vi "Save Bar Sample test results to Disk.vi"(0 "Test Settings":T4={"Current Level"=0.0, "Compliance Level"=0.0, "Soak Time"=0.0, "NPLC Voltmeter"=1.0, "Count Voltmeter"=1, "NPLC Ammeter"=1.0, "Count Ammeter"=1, "Sample Resistivity"=enum."Low", "Sample Thickness"=0.0, "Magnetic Flux"=0.0, "Units"=enum."T", "Sample Dimensions x"=0.0, "Sample Dimensions y"=0.0, "Sample Dimensions D1"=0.0, "Sample Dimensions D2"=0.0, "Sample Width Ws"=0.0, "Slot Number of 3765 card"=1} {"Slot Number of 3765 card" min=1 max=6; "NPLC Ammeter" min=0.01 max=10.0; "NPLC Voltmeter" min=0.01 max=10.0 format="%^#_6g"; "Count Ammeter" min=1 max=1024; "Count Voltmeter" min=1 max=1024; "Soak Time" format="%^#_6g"; "Compliance Level" format="%^#_6g"; "Current Level" format="%^#_6e"}, 1 "Sample Name":string, 2 "User Name":string, 3 "Test Date":string, 5 "Bar Sample Measurements":T2, 7 "Bar Sample Results":T1, 11 "error in (no error)":errorcluster, 12 "Save To Path":path) -> (15 "error out":errorcluster)   [LabVIEW 2016]
uses:
  Hall Effect Library/Public/Controls/Resisitivity.ctl
  Hall Effect Library/Hall Effect Library.lvlib
panel:
  # "Carrier Concentration"
  # "p"
  # "Vr"
  # "Vh"
  # "NPLC"
  # "A"
  # "V"
  # "s"
  # "Measure Count"
  # "cm"
  # "cm"
  # "cm"
  # "cm"
  # "cm"
  # "cm"
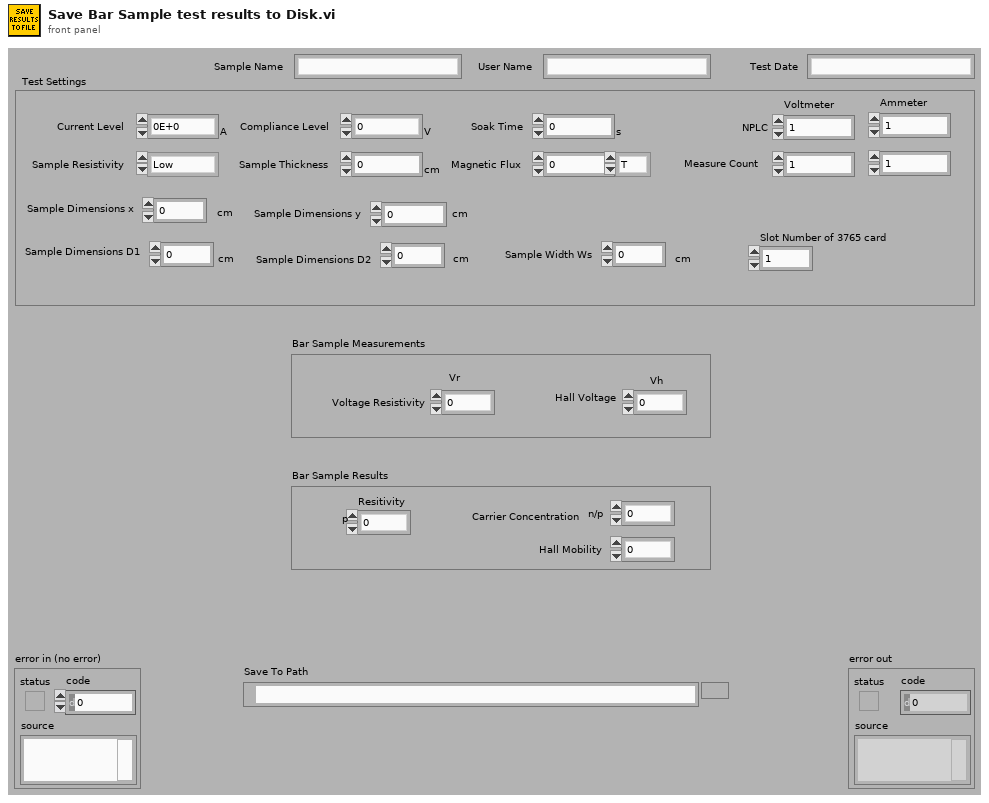
[diagram p1: front panel]
types:
  T1 = cluster{"Resitivity":dbl, "n/p":dbl, "Hall Mobility":dbl}
  T2 = cluster{"Voltage Resistivity":dbl, "Hall Voltage":dbl}
  T3 = typedef "Hall Effect Library.lvlib/Resisitivity.ctl" = enum16{"Low", "High"}
  T4 = cluster{"Current Level":dbl, "Compliance Level":dbl, "Soak Time":dbl, "NPLC Voltmeter":dbl, "Count Voltmeter":i32, "NPLC Ammeter":dbl, "Count Ammeter":i32, "Sample Resistivity":T3, "Sample Thickness":dbl, "Magnetic Flux":dbl, "Units":enum16{"Gs", "T"}, "Sample Dimensions x":dbl, "Sample Dimensions y":dbl, "Sample Dimensions D1":dbl, "Sample Dimensions D2":dbl, "Sample Width Ws":dbl, "Slot Number of 3765 card":u16}
  T5 = enum16{"open", "replace", "create", "open or create", "replace or create", "replace or create with confirmation"}
  T6 = cluster{"Bar Sample Resistivity Currents[0]":dbl}
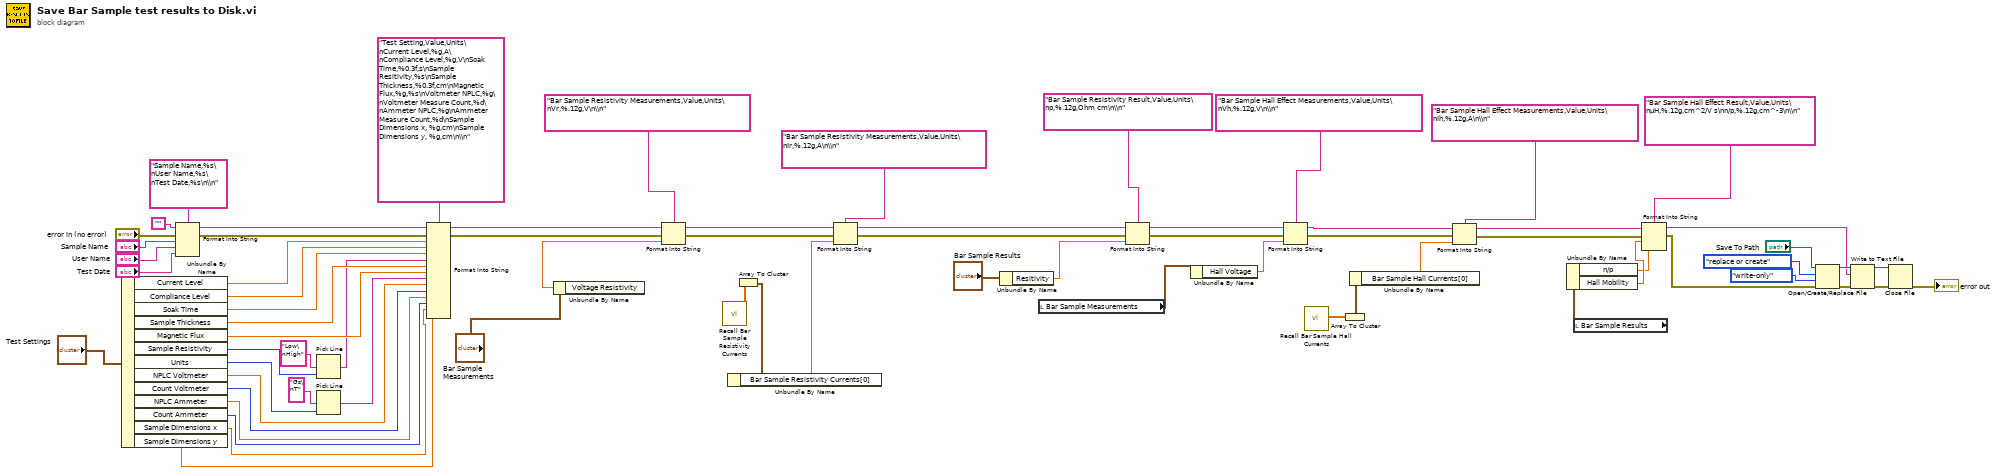
[diagram p0: block diagram]
diagram:
  n1 = Unbundle By Name("Test Settings") -> ("Current Level"=w63:dbl, "Compliance Level"=w62:dbl, "Soak Time"=w61:dbl, "Sample Thickness"=w60:dbl, "Magnetic Flux"=w59:dbl, "Sample Resistivity"=w55:T3, "Units"=w56:enum16{"Gs", "T"}, "NPLC Voltmeter"=w31:dbl, "Count Voltmeter"=w30:i32, "NPLC Ammeter"=w29:dbl, "Count Ammeter"=w28:i32, "Sample Dimensions x"=w27:dbl, "Sample Dimensions y"=w26:dbl)
  n2 = Format Into String(format string="Sample Name,%s\nUser Name,%s\nTest Date,%s\n\\n", initial string="", error in="error in (no error)", "Sample Name", "User Name", "Test Date") -> (resulting string=w51:string, error out=w52:errorcluster)
  n3 = Pick Line(multi-line string="Low\nHigh", line index=w55) -> (output string=w54:string)  [unwired: 1 out]
  n4 = Pick Line(multi-line string="Gs\nT", line index=w56) -> (output string=w53:string)  [unwired: 1 out]
  n5 = Format Into String(format string="Test Setting,Value,Units\nCurrent Level,%g,A\nCompliance Level,%g,V\nSoak Time,%0.3f,s\nSample Resitivity,%s\nSample Thickness,%0.3f,cm\nMagnetic Flux,%g,%s\nVoltmeter NPLC,%g\nVoltmeter Measure Count,%d\nAmmeter NPLC,%g\nAmmeter Measure Count,%d\nSample Dimensions x, %g,cm\nSample Dimensions y, %g,cm\n\\n", initial string=w51, error in=w52, w63, w62, w61, w54, w60, w59, w53, w31, w30, w29, w28, w27, w26) -> (resulting string=w49:string, error out=w48:errorcluster)
  n6 = Unbundle By Name("Bar Sample Measurements") -> ("Voltage Resistivity"=w24:dbl)
  n7 = Format Into String(format string="Bar Sample Resistivity Measurements,Value,Units\nVr,%.12g,V\n\\n", initial string=w49, error in=w48, w24) -> (resulting string=w12:string, error out=w13:errorcluster)
  n8 = call "Recall Bar Sample Resistivity Currents.vi"() -> ("Bar Sample Resistivity Currents"=w16:dbl[])  [unwired: 11 in]
  n9 = Array To Cluster(array=w16) -> (cluster=w15:T6)
  n10 = Unbundle By Name(w15) -> ("Bar Sample Resistivity Currents[0]"=w14:dbl)
  n11 = Format Into String(format string="Bar Sample Resistivity Measurements,Value,Units\nIr,%.12g,A\n\\n", initial string=w12, error in=w13, w14) -> (resulting string=w10:string, error out=w9:errorcluster)
  n12 = Unbundle By Name("Bar Sample Results") -> ("Resitivity"=w22:dbl)
  n13 = local read "Bar Sample Measurements"() -> (w21:T2)
  n14 = Format Into String(format string="Bar Sample Resistivity Result,Value,Units\np,%.12g,Ohm cm\n\\n", initial string=w10, error in=w9, w22) -> (resulting string=w45:string, error out=w44:errorcluster)
  n15 = Unbundle By Name(w21) -> ("Hall Voltage"=w20:dbl)
  n16 = Format Into String(format string="Bar Sample Hall Effect Measurements,Value,Units\nVh,%.12g,V\n\\n", initial string=w45, error in=w44, w20) -> (resulting string=w5:string, error out=w4:errorcluster)
  n17 = call "Recall Bar Sample Hall Currents.vi"() -> ("Bar Sample Hall Currents"=w8:dbl[])  [unwired: 11 in]
  n18 = Array To Cluster(array=w8) -> (cluster=w7:cluster{"Bar Sample Hall Currents[0]":dbl})
  n19 = Unbundle By Name(w7) -> ("Bar Sample Hall Currents[0]"=w6:dbl)
  n20 = Format Into String(format string="Bar Sample Hall Effect Measurements,Value,Units\nIh,%.12g,A\n\\n", initial string=w5, error in=w4, w6) -> (resulting string=w3:string, error out=w2:errorcluster)
  n21 = local read "Bar Sample Results"() -> (w19:T1)
  n22 = Unbundle By Name(w19) -> ("n/p"=w17:dbl, "Hall Mobility"=w18:dbl)
  n23 = Format Into String(format string="Bar Sample Hall Effect Result,Value,Units\nµH,%.12g,cm^2/V s\nn/p,%.12g,cm^-3\n\\n", initial string=w3, error in=w2, w18, w17) -> (resulting string=w34:string, error out=w35:errorcluster)
  n24 = Open/Create/Replace File(file path (use dialog)="Save To Path", error in=w35, operation (0:open)=T5."replace or create", access (0:read/write)=enum16{"read/write", "read-only", "write-only"}."write-only") -> (refnum out=w39:refnum<file>, error out=w38:errorcluster)  [unwired: 3 out]
  n25 = Write to Text File(file (use dialog)=w39, text=w34, error in=w38) -> (refnum out=w36:refnum<file>, error out=w37:errorcluster)  [unwired: 2 out]
  n26 = Close File(refnum=w36, error in=w37) -> (error out=→"error out":errorcluster)  [unwired: 1 out]
